vi "list.get.vi"(8 "error in":errorcluster, 10 "index":i32, 11 "List in":refnum<class "List.lvclass">) -> (0 "error out":errorcluster, 2 "handle":i32, 3 "List out":refnum<class "List.lvclass">)   [LabVIEW 2020, in "List.lvclass"]
uses:
  List.lvclass
  List.lvclass/List.ctl
  client.lvlib
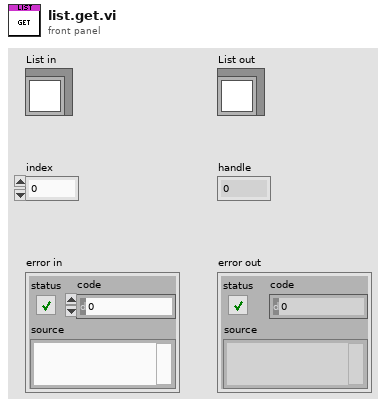
[diagram p1: front panel]
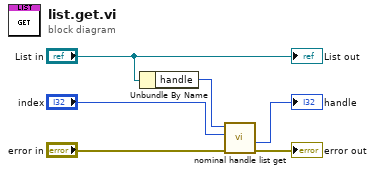
[diagram p0: block diagram]
diagram:
  n1 = Unbundle By Name("List in") -> ("handle"=w2:i32)
  n2 = call "nominal handle list get.vi"("error in (no error)"="error in", "index"="index", "list"=w2) -> ("error out"=→"error out":errorcluster, "out_handle out"=→"handle":i32)  [unwired: 6 in, 1 out]
  "List out" <- "List in"
